vi "write_sample_weight.vi"(8 "error in (no error)":errorcluster, 10 "sample_weight":dbl[](array[numeric]), 11 "LassoLarsCV in":refnum<class "LassoLarsCV.lvclass">) -> (0 "error out":errorcluster, 3 "LassoLarsCV out":refnum<class "LassoLarsCV.lvclass">)   [LabVIEW 2020, in "LassoLarsCV.lvclass"]
uses:
  LassoLarsCV.lvclass
  LassoLarsCV.lvclass/LassoLarsCV.ctl
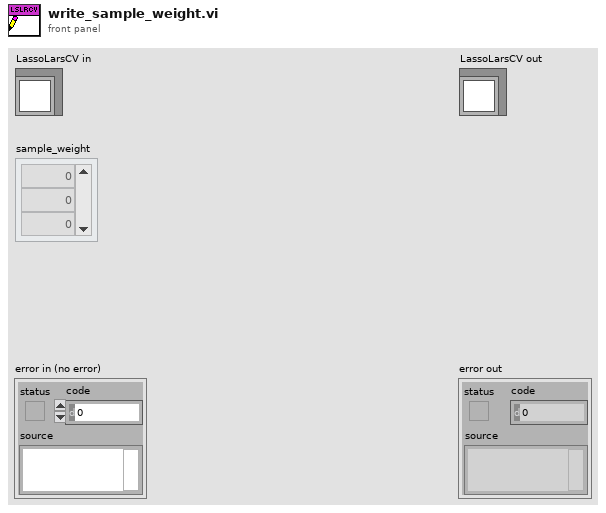
[diagram p1: front panel]
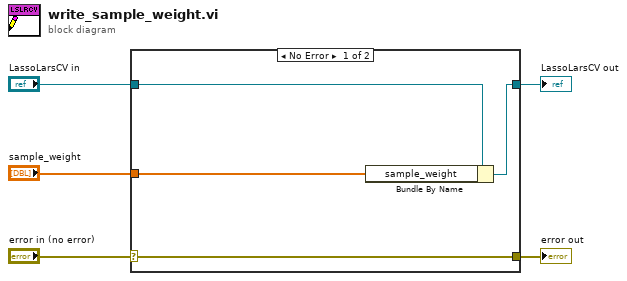
[diagram p0: block diagram]
diagram:
  n1 = case shown="No Error" "error in (no error)" {
    selector: "error in (no error)" -> [w9 w10]
    tunnel: [w9 w10] -> w4
    tunnel: [w7 w11] -> w2
    tunnel: "LassoLarsCV in" -> [w8 w11]
    tunnel: "sample_weight" -> [w6 _]
    frame No Error {
      n2 = Bundle By Name(cluster=w8, "sample_weight"=w6) -> (w7:refnum<class "LassoLarsCV.lvclass">)
    }
    frame Error {
    }
  }
  "error out" <- w4
  "LassoLarsCV out" <- w2
